vi "加密解密字符串（XOR）.vi"(8 "error in (no error)":errorcluster caption="错误输入（无错误）", 9 "密钥":u8=30, 11 "输入字符串":string) -> (0 "error out":errorcluster caption="错误输出", 3 "输出字符串":string)   [LabVIEW 2012]
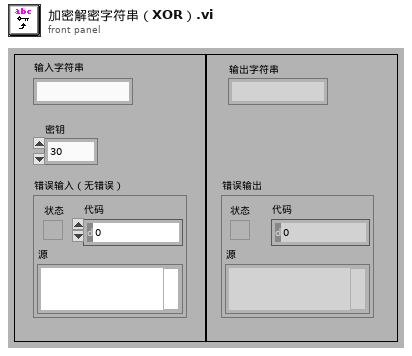
[diagram p1: front panel]
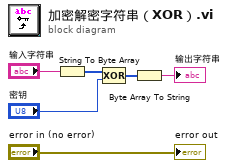
[diagram p0: block diagram]
diagram:
  n1 = String To Byte Array(string="输入字符串") -> (unsigned byte array=w5:u8[])
  n2 = Compound Arithmetic op=XOR(w5, "密钥") -> (w4:u8[])
  n3 = Byte Array To String(unsigned byte array=w4) -> (string=→"输出字符串":string)
  "error out" <- "error in (no error)"
